vi "VISA_Scan.vi"(8 "error in (no error)":errorcluster, 11 "DataCluster":T1={"Core"={"Current VI Reference"=refnum, "Close Panel on Exit?"=FALSE, "Exit"=FALSE, "Initialized?"=FALSE}, "Connections"={"cDAQ"={"Task"="", "Connected"=FALSE, "Active"=FALSE, "ID"=""}, "Camera"={"Session"="", "Connected"=FALSE, "Active"=FALSE, "Placeholder"=refnum}, "PSU"={"Port"="", "Connected"=FALSE, "Active"=FALSE}, "Arduino"={"Port"="", "Connected"=FALSE, "Active"=FALSE}}, "Data Acquisition"={"Setup"={"Label"="", "Operator"="", "Notes"="", "TempGrad"=0.0, "TargetTemp"=0.0, "Sample Volume"=1.0}, "Camera"={"Image"=refnum, "Save Image"=refnum, "Image Frequency"=20, "Rectangle"={"Left"=0, "Top"=0, "Right"=0, "Bottom"=0, "Rotation"=0.0}, "Calibration"={"Top Left"={"X"=0.0, "Y"=0.0}, "Top Right"={"X"=0.0, "Y"=0.0}, "Bottom Left"={"X"=0.0, "Y"=0.0}, "Bottom Right"={"X"=0.0, "Y"=0.0}, "Fixpoint"={"X"=0.0, "Y"=0.0}, "Scan Area"=0.0, "Fixpoint Area"=0.0, "Well Pixels"=[], "Valid"=FALSE}, "FocusPos"=0, "Display Mapping"=10, "Camera Mode"=10}, "Thermistor"={"Sample Size"=0, "Calibration"={"B0.100"=[], "R25"=[], "c"=[], "State"=[], "V_S"=0.0, "R_S"=0.0}, "Timing Mode"=14713}, "Partition"={"Data"=[], "Cell Label"="", "Cell Color"=0, "Height"=10, "Width"=16, "Grid"=[]}, "Queue"={"Size"=0, "Queue"=refnum}, "Sample Rate"=0, "Active"=FALSE, "Ready"=FALSE, "Graph Mode"=0, "Gradient Buffer"=2}, "Control"={"Sample Rate"=0, "PID gains"={"proportional gain (Kc)"=0.0, "integral time (Ti, min)"=0.0, "derivative time (Td, min)"=0.0}}, "Manual Temp Control"={"TargetTemp"=1.0, "Mode"=0, "Active"=FALSE}} {"Manual Temp Control"."Mode" items=["Cool", "Heat"]; "Manual Temp Control"."TargetTemp" min=-40.0 max=40.0 step=0.5 format="%#_g °C"; "Control"."PID gains"."derivative time (Td, min)" format="%.3f"; "Control"."PID gains"."integral time (Ti, min)" format="%.3f"; "Control"."PID gains"."proportional gain (Kc)" format="%.3f"; "Control"."Sample Rate" min=1 max=20 step=1 format="%.0f Samples/sec"; "Data Acquisition"."Gradient Buffer" min=2 max=30 step=1; "Data Acquisition"."Graph Mode" items=["Thermistor Temperature", "Camera Temperature"]; "Data Acquisition"."Thermistor"."Timing Mode" items=["Automatic"=16097, "High Resolution"=10195, "High Speed"=14712, "Best 50 Hz Rejection"=14713, "Best 60 Hz Rejection"=14714, "Custom"=10137]; "Data Acquisition"."Thermistor"."Calibration"."R_S" min=0.1 max=1000.0 format="%#_g kOhm"; "Data Acquisition"."Thermistor"."Calibration"."V_S" min=5.0 max=48.0 format="%#_g V"; "Data Acquisition"."Thermistor"."Calibration"."R25" min=0.1 max=1000.0 format="%#_g kOhm"; "Data Acquisition"."Thermistor"."Calibration"."B0.100" min=100.0 max=10000.0 format="%#_g K"; "Data Acquisition"."Thermistor"."Sample Size" min=1 max=200; "Data Acquisition"."Sample Rate" min=20 max=240 format="%.0f samples/min"; "Data Acquisition"."Queue"."Size" min=1 max=200; "Data Acquisition"."Camera"."Camera Mode" items=["Temperature Linear", "Signal Linear"]; "Data Acquisition"."Camera"."Display Mapping" items=["Default"=10, "Most Significant Bits"=11, "Full Dynamic"=12, "Downshift"=13, "Given Range"=14, "90% Dynamic"=15, "Given Percent Range"=16]; "Data Acquisition"."Camera"."Calibration"."Fixpoint"."Y" format="%.2f"; "Data Acquisition"."Camera"."Calibration"."Fixpoint"."X" format="%.2f"; "Data Acquisition"."Camera"."Calibration"."Top Left"."Y" format="%.2f"; "Data Acquisition"."Camera"."Calibration"."Top Left"."X" format="%.2f"; "Data Acquisition"."Camera"."Calibration"."Top Right"."Y" format="%.2f"; "Data Acquisition"."Camera"."Calibration"."Top Right"."X" format="%.2f"; "Data Acquisition"."Camera"."Calibration"."Bottom Left"."Y" format="%.2f"; "Data Acquisition"."Camera"."Calibration"."Bottom Left"."X" format="%.2f"; "Data Acquisition"."Camera"."Calibration"."Bottom Right"."Y" format="%.2f"; "Data Acquisition"."Camera"."Calibration"."Bottom Right"."X" format="%.2f"; "Data Acquisition"."Camera"."Rectangle"."Rotation" min=-90.0 max=90.0 step=1.0 format="%.2f"; "Data Acquisition"."Camera"."Rectangle"."Left" scale=0.0..1024.0; "Data Acquisition"."Camera"."Rectangle"."Right" scale=0.0..1024.0; "Data Acquisition"."Camera"."Image Frequency" min=1 max=60 step=1; "Data Acquisition"."Setup"."Sample Volume" min=0.0 max=500.0 format="%#_g µL"; "Data Acquisition"."Setup"."TargetTemp" min=-40.0 max=40.0 step=0.5 format="%#_g °C"; "Data Acquisition"."Setup"."TempGrad" min=-100.0 max=100.0 step=0.1 format="%#_g °C/min"}) -> (0 "error out":errorcluster, 1 "State out":string, 2 "Connected?":bool, 3 "DataCluster out":T1={"Core"={"Current VI Reference"=refnum, "Close Panel on Exit?"=FALSE, "Exit"=FALSE, "Initialized?"=FALSE}, "Connections"={"cDAQ"={"Task"="", "Connected"=FALSE, "Active"=FALSE, "ID"=""}, "Camera"={"Session"="", "Connected"=FALSE, "Active"=FALSE, "Placeholder"=refnum}, "PSU"={"Port"="", "Connected"=FALSE, "Active"=FALSE}, "Arduino"={"Port"="", "Connected"=FALSE, "Active"=FALSE}}, "Data Acquisition"={"Setup"={"Label"="", "Operator"="", "Notes"="", "TempGrad"=1.0, "TargetTemp"=1.0, "Sample Volume"=1.0}, "Camera"={"Image"=refnum, "Save Image"=refnum, "Image Frequency"=20, "Rectangle"={"Left"=0, "Top"=0, "Right"=0, "Bottom"=0, "Rotation"=0.0}, "Calibration"={"Top Left"={"X"=0.0, "Y"=0.0}, "Top Right"={"X"=0.0, "Y"=0.0}, "Bottom Left"={"X"=0.0, "Y"=0.0}, "Bottom Right"={"X"=0.0, "Y"=0.0}, "Fixpoint"={"X"=0.0, "Y"=0.0}, "Scan Area"=0.0, "Fixpoint Area"=0.0, "Well Pixels"=[], "Valid"=FALSE}, "FocusPos"=0, "Display Mapping"=10, "Camera Mode"=10}, "Thermistor"={"Sample Size"=1, "Calibration"={"B0.100"=[], "R25"=[], "c"=[], "State"=[], "V_S"=5.0, "R_S"=100.0}, "Timing Mode"=14713}, "Partition"={"Data"=[], "Cell Label"="", "Cell Color"=0, "Height"=10, "Width"=16, "Grid"=[]}, "Queue"={"Size"=1, "Queue"=refnum}, "Sample Rate"=20, "Active"=FALSE, "Ready"=FALSE, "Graph Mode"=0, "Gradient Buffer"=2}, "Control"={"Sample Rate"=1, "PID gains"={"proportional gain (Kc)"=1.0, "integral time (Ti, min)"=0.01, "derivative time (Td, min)"=0.0}}, "Manual Temp Control"={"TargetTemp"=1.0, "Mode"=0, "Active"=FALSE}} {"Manual Temp Control"."Mode" items=["Cool", "Heat"]; "Manual Temp Control"."TargetTemp" min=-40.0 max=40.0 step=0.5 format="%#_g °C"; "Control"."PID gains"."derivative time (Td, min)" format="%.3f"; "Control"."PID gains"."integral time (Ti, min)" format="%.3f"; "Control"."PID gains"."proportional gain (Kc)" format="%.3f"; "Control"."Sample Rate" min=1 max=20 step=1 format="%.0f Samples/sec"; "Data Acquisition"."Gradient Buffer" min=2 max=30 step=1; "Data Acquisition"."Graph Mode" items=["Thermistor Temperature", "Camera Temperature"]; "Data Acquisition"."Thermistor"."Timing Mode" items=["Automatic"=16097, "High Resolution"=10195, "High Speed"=14712, "Best 50 Hz Rejection"=14713, "Best 60 Hz Rejection"=14714, "Custom"=10137]; "Data Acquisition"."Thermistor"."Calibration"."R_S" min=0.1 max=1000.0 format="%#_g kOhm"; "Data Acquisition"."Thermistor"."Calibration"."V_S" min=5.0 max=48.0 format="%#_g V"; "Data Acquisition"."Thermistor"."Calibration"."R25" min=0.1 max=1000.0 format="%#_g kOhm"; "Data Acquisition"."Thermistor"."Calibration"."B0.100" min=100.0 max=10000.0 format="%#_g K"; "Data Acquisition"."Thermistor"."Sample Size" min=1 max=200; "Data Acquisition"."Sample Rate" min=20 max=240 format="%.0f samples/min"; "Data Acquisition"."Queue"."Size" min=1 max=200; "Data Acquisition"."Camera"."Camera Mode" items=["Temperature Linear", "Signal Linear"]; "Data Acquisition"."Camera"."Display Mapping" items=["Default"=10, "Most Significant Bits"=11, "Full Dynamic"=12, "Downshift"=13, "Given Range"=14, "90% Dynamic"=15, "Given Percent Range"=16]; "Data Acquisition"."Camera"."Calibration"."Fixpoint"."Y" format="%.2f"; "Data Acquisition"."Camera"."Calibration"."Fixpoint"."X" format="%.2f"; "Data Acquisition"."Camera"."Calibration"."Top Left"."Y" format="%.2f"; "Data Acquisition"."Camera"."Calibration"."Top Left"."X" format="%.2f"; "Data Acquisition"."Camera"."Calibration"."Top Right"."Y" format="%.2f"; "Data Acquisition"."Camera"."Calibration"."Top Right"."X" format="%.2f"; "Data Acquisition"."Camera"."Calibration"."Bottom Left"."Y" format="%.2f"; "Data Acquisition"."Camera"."Calibration"."Bottom Left"."X" format="%.2f"; "Data Acquisition"."Camera"."Calibration"."Bottom Right"."Y" format="%.2f"; "Data Acquisition"."Camera"."Calibration"."Bottom Right"."X" format="%.2f"; "Data Acquisition"."Camera"."Rectangle"."Rotation" min=-90.0 max=90.0 step=1.0 format="%.2f"; "Data Acquisition"."Camera"."Rectangle"."Left" scale=0.0..1024.0; "Data Acquisition"."Camera"."Rectangle"."Right" scale=0.0..1024.0; "Data Acquisition"."Camera"."Image Frequency" min=1 max=60 step=1; "Data Acquisition"."Setup"."Sample Volume" min=0.0 max=500.0 format="%#_g µL"; "Data Acquisition"."Setup"."TargetTemp" min=-40.0 max=40.0 step=0.5 format="%#_g °C"; "Data Acquisition"."Setup"."TempGrad" min=-100.0 max=100.0 step=0.1 format="%#_g °C/min"})   [LabVIEW 2024]
uses:
  DataCluster.ctl
  <vilib>/userDefined/High Color/IMAQdx.ctl
  <vilib>/vision/Image Controls.llb/IMAQ Image.ctl
  b3916838-8fe5-48f2-9af3-802836062305.vi
  05927bd2-cd8c-4d85-a005-f947e7e15427.vi
  d6bb83c9-de94-4caf-9b41-0debf6542286.vi
  <vilib>/regexp/Match Regular Expression.xnode
panel:
  out "Interface Description":string
  out "find list":string[](array[string])
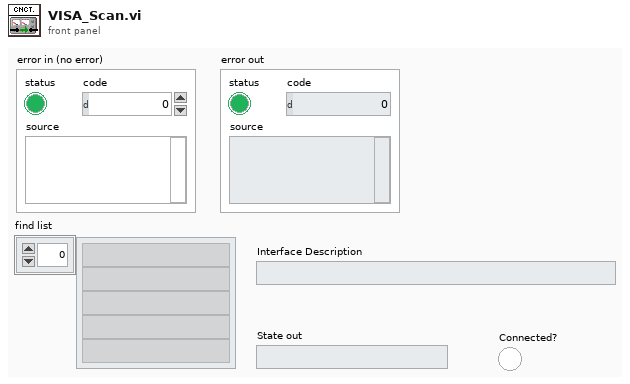
[diagram p1: front panel]
types:
  T1 = typedef "DataCluster.ctl" = cluster{"Core":cluster{"Current VI Reference":refnum<vi>, "Close Panel on Exit?":bool, "Exit":bool, "Initialized?":bool}, "Connections":cluster{"cDAQ":cluster{"Task":refnum<k21>, "Connected":bool, "Active":bool, "ID":string}, "Camera":cluster{"Session":T2, "Connected":bool, "Active":bool, "Placeholder":T3}, "PSU":cluster{"Port":refnum<visa-resource-name>, "Connected":bool, "Active":bool}, "Arduino":cluster{"Port":refnum<visa-resource-name>, "Connected":bool, "Active":bool}}, "Data Acquisition":cluster{"Setup":cluster{"Label":string, "Operator":string, "Notes":string, "TempGrad":dbl, "TargetTemp":dbl, "Sample Volume":dbl}, "Camera":cluster{"Image":T3, "Save Image":T3, "Image Frequency":i32, "Rectangle":T4, "Calibration":cluster{"Top Left":T5, "Top Right":T5, "Bottom Left":T5, "Bottom Right":T5, "Fixpoint":T5, "Scan Area":dbl, "Fixpoint Area":dbl, "Well Pixels":cluster{"X":i32, "Y":i32}[][], "Valid":bool}, "FocusPos":u32, "Display Mapping":u32, "Camera Mode":u32}, "Thermistor":cluster{"Sample Size":i32, "Calibration":cluster{"B0.100":dbl[], "R25":dbl[], "c":dbl[][], "State":bool[], "V_S":dbl, "R_S":dbl}, "Timing Mode":i32}, "Partition":cluster{"Data":string[][], "Cell Label":string, "Cell Color":u32, "Height":i32, "Width":i32, "Grid":string[][]}, "Queue":cluster{"Size":i32, "Queue":refnum<queue>}, "Sample Rate":i32, "Active":bool, "Ready":bool, "Graph Mode":u16, "Gradient Buffer":i32}, "Control":cluster{"Sample Rate":i32, "PID gains":cluster{"proportional gain (Kc)":dbl, "integral time (Ti, min)":dbl, "derivative time (Td, min)":dbl}}, "Manual Temp Control":cluster{"TargetTemp":dbl, "Mode":u16, "Active":bool}}
  T2 = typedef "IMAQdx.ctl" = refnum<k21>
  T3 = typedef "IMAQ Image.ctl" = refnum<image>
  T4 = typedef "IMAQ Rectangle" = cluster{"Left":i32, "Top":i32, "Right":i32, "Bottom":i32, "Rotation":dbl}
  T5 = typedef "IMAQ Point" = cluster{"X":sgl, "Y":sgl}
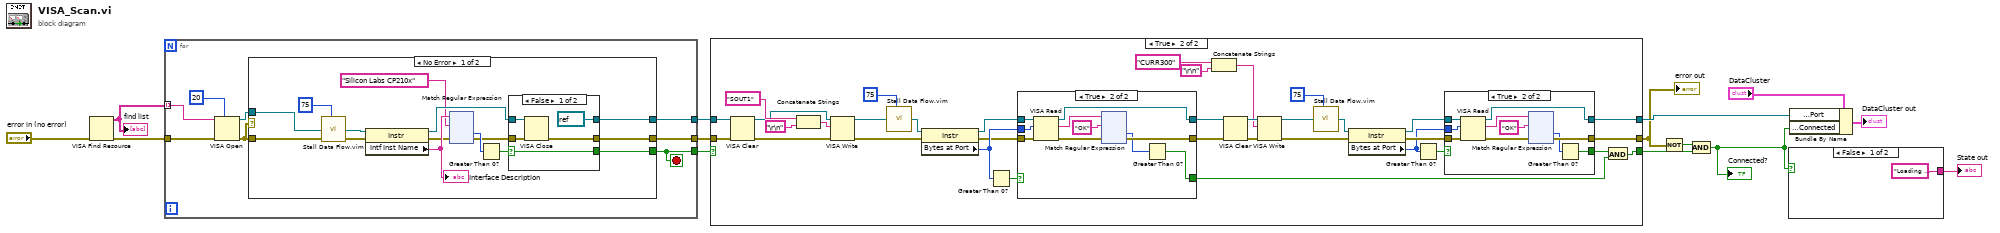
[diagram p0: block diagram]
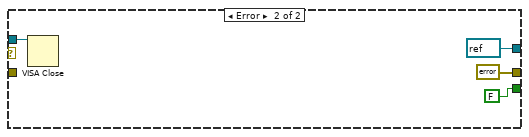
[diagram p4: hidden frame]
diagram:
  n1 = VISA Find Resource(8:"error in (no error)") -> (0:w13:errorcluster, 3:w14:string[])  [unwired: 2 in, 1 out]
  "find list" <- w14
  n2 = for {
    tunnel: w14 -> [w22] mode=indexing
    tunnel: w13 -> [w21]
    tunnel: [w18] -> w9
    tunnel: [w17] -> w11
    tunnel: [w19] -> w10
    stop <- w17 stop-if-true
    n3 = VISA Open(timeout (0)=u32 20 ("VISA Open timeout (0)"), error in (no error)=w21, VISA resource name=w22) -> (VISA resource name=w16:refnum<visa-resource-name>, error out=w20:errorcluster)  [unwired: 2 in]
    n4 = case shown="No Error" w20 {
      tunnel: w16 -> [w25 w163]
      tunnel: w20 -> [w36 _]
      tunnel: [w32 refnum<visa-resource-name> refnum ("Port")] -> w19
      tunnel: [w31 FALSE] -> w17
      tunnel: [w30 errorcluster {"status"=FALSE, "code"=0, "source"=""} ("error out")] -> w18
      frame No Error {
        n5 = call "Stall Data Flow.vim"("value in"=w25, "milliseconds to wait"=u32 75) -> ("value out"=w24:refnum<visa-resource-name>)  [unwired: 1 out]
        n6 = property class="Instr"(reference=w24, error in=w36) -> (reference out=w33:refnum<visa-resource-name>, error out=w27:errorcluster, "Intf Inst Name"=w35:string)
        "Interface Description" <- w35
        n7 = xnode "Match Regular Expression"("input string"=w35, "regular expression"="Silicon Labs CP210x", "error in"=w27) -> ("offset past match"=w28:i32, "error out"=w26:errorcluster)  [unwired: 3 in, 3 out]
        n8 = Greater Than 0?(x=w28) -> (x > 0?=w34:bool)
        n9 = case shown="False" w34 {
          selector: w34 -> [w158 w160]
          tunnel: w33 -> [w157 w161]
          tunnel: [refnum<visa-resource-name> refnum ("Port") w161] -> w32
          tunnel: [w158 w160] -> w31
          tunnel: w26 -> [w156 w159]
          tunnel: [w155 w159] -> w30
          frame False {
            n10 = VISA Close(VISA resource name=w157, error in (no error)=w156) -> (error out=w155:errorcluster)
          }
          frame True {
          }
        }
      }
      frame Error {
        n11 = VISA Close(VISA resource name=w163) -> ()  [unwired: 1 in, 1 out]
      }
    }
  }
  n12 = case shown="True" w11 {
    selector: w11 -> [w167 _]
    tunnel: w10 -> [w166 w200]
    tunnel: w9 -> [w168 w199]
    tunnel: [w166 w171] -> w7
    tunnel: [w168 w172] -> w3
    tunnel: [w167 w170] -> w5
    frame False {
    }
    frame True {
      n13 = VISA Clear(VISA resource name=w200, error in (no error)=w199) -> (VISA resource name out=w198:refnum<visa-resource-name>, error out=w197:errorcluster)
      n14 = Concatenate Strings("SOUT1" ("string"), "\r\n") -> (w201:string)
      n15 = VISA Write(VISA resource name=w198, write buffer=w201, error in (no error)=w197) -> (VISA resource name out=w190:refnum<visa-resource-name>, error out=w189:errorcluster)  [unwired: 1 out]
      n16 = call "Stall Data Flow.vim"("value in"=w190, "milliseconds to wait"=u32 75) -> ("value out"=w196:refnum<visa-resource-name>)  [unwired: 1 out]
      n17 = property class="Instr"(reference=w196, error in=w189) -> (reference out=w193:refnum<visa-resource-name>, error out=w192:errorcluster, "Bytes at Port"=w194:u32)
      n18 = Greater Than 0?(x=w194) -> (x > 0?=w195:bool)
      n19 = case shown="True" w195 {
        selector: w195 -> [w334 _]
        tunnel: w194 -> [_ w346]
        tunnel: w192 -> [w335 w345]
        tunnel: [w336 w344] -> w174
        tunnel: [w335 w339] -> w173
        tunnel: w193 -> [w336 w343]
        tunnel: [w334 w337] -> w188
        frame False {
        }
        frame True {
          n20 = VISA Read(VISA resource name=w343, byte count=w346, error in (no error)=w345) -> (VISA resource name out=w344:refnum<visa-resource-name>, read buffer=w342:string, error out=w341:errorcluster)  [unwired: 1 out]
          n21 = xnode "Match Regular Expression"("input string"=w342, "regular expression"="OK", "error in"=w341) -> ("offset past match"=w338:i32, "error out"=w339:errorcluster)  [unwired: 3 in, 3 out]
          n22 = Greater Than 0?(x=w338) -> (x > 0?=w337:bool)
        }
      }
      n23 = Concatenate Strings("CURR300" ("string"), "\r\n") -> (w178:string)
      n24 = VISA Clear(VISA resource name=w174, error in (no error)=w173) -> (VISA resource name out=w179:refnum<visa-resource-name>, error out=w180:errorcluster)
      n25 = VISA Write(VISA resource name=w179, write buffer=w178, error in (no error)=w180) -> (VISA resource name out=w186:refnum<visa-resource-name>, error out=w187:errorcluster)  [unwired: 1 out]
      n26 = call "Stall Data Flow.vim"("value in"=w186, "milliseconds to wait"=u32 75) -> ("value out"=w181:refnum<visa-resource-name>)  [unwired: 1 out]
      n27 = property class="Instr"(reference=w181, error in=w187) -> (reference out=w184:refnum<visa-resource-name>, error out=w185:errorcluster, "Bytes at Port"=w183:u32)
      n28 = Greater Than 0?(x=w183) -> (x > 0?=w182:bool)
      n29 = case shown="True" w182 {
        selector: w182 -> [w204 _]
        tunnel: w183 -> [_ w216]
        tunnel: w185 -> [w205 w215]
        tunnel: [w206 w214] -> w171
        tunnel: [w205 w209] -> w172
        tunnel: w184 -> [w206 w213]
        tunnel: [w204 w207] -> w169
        frame False {
        }
        frame True {
          n30 = VISA Read(VISA resource name=w213, byte count=w216, error in (no error)=w215) -> (VISA resource name out=w214:refnum<visa-resource-name>, read buffer=w212:string, error out=w211:errorcluster)  [unwired: 1 out]
          n31 = xnode "Match Regular Expression"("input string"=w212, "regular expression"="OK", "error in"=w211) -> ("offset past match"=w208:i32, "error out"=w209:errorcluster)  [unwired: 3 in, 3 out]
          n32 = Greater Than 0?(x=w208) -> (x > 0?=w207:bool)
        }
      }
      n33 = And(x=w169, y=w188) -> (x .and. y?=w170:bool)
    }
  }
  "error out" <- w3
  n34 = Not(x=w3) -> (.not. x?=w1:bool)
  n35 = And(x=w1, y=w5) -> (x .and. y?=w2:bool)
  "Connected?" <- w2
  n36 = case shown="False" w2 {
    tunnel: ["Loading UI: Description >> PSU Connection Failed!" _] -> w4
    frame False {
    }
    frame True {
    }
  }
  "State out" <- w4
  n37 = Bundle By Name(cluster="DataCluster", "Connections.PSU.Port"=w7, "Connections.PSU.Connected"=w2) -> (→"DataCluster out":T1)
